vi "Blink_SDK_example_ODP.vi"() -> ()   [LabVIEW 2010]
uses:
  Blink_C_wrapper.dll
  ImageGen.dll
panel:
  in  "True frames":i64=5
  in  "SLM bit depth":u64=8
  out "Boards found":u64
  out "Constructed OK":i64
  in  "Use GPU if available":i64=1
  in  "Maximum Transient Frames":i64=10
  out "Regional LUT File":path
  # "SLM Settings"
  # "These settings should be changed to match your SLM\nbefore running the program."
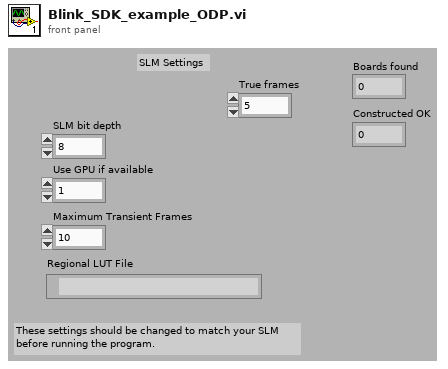
[diagram p1: front panel]
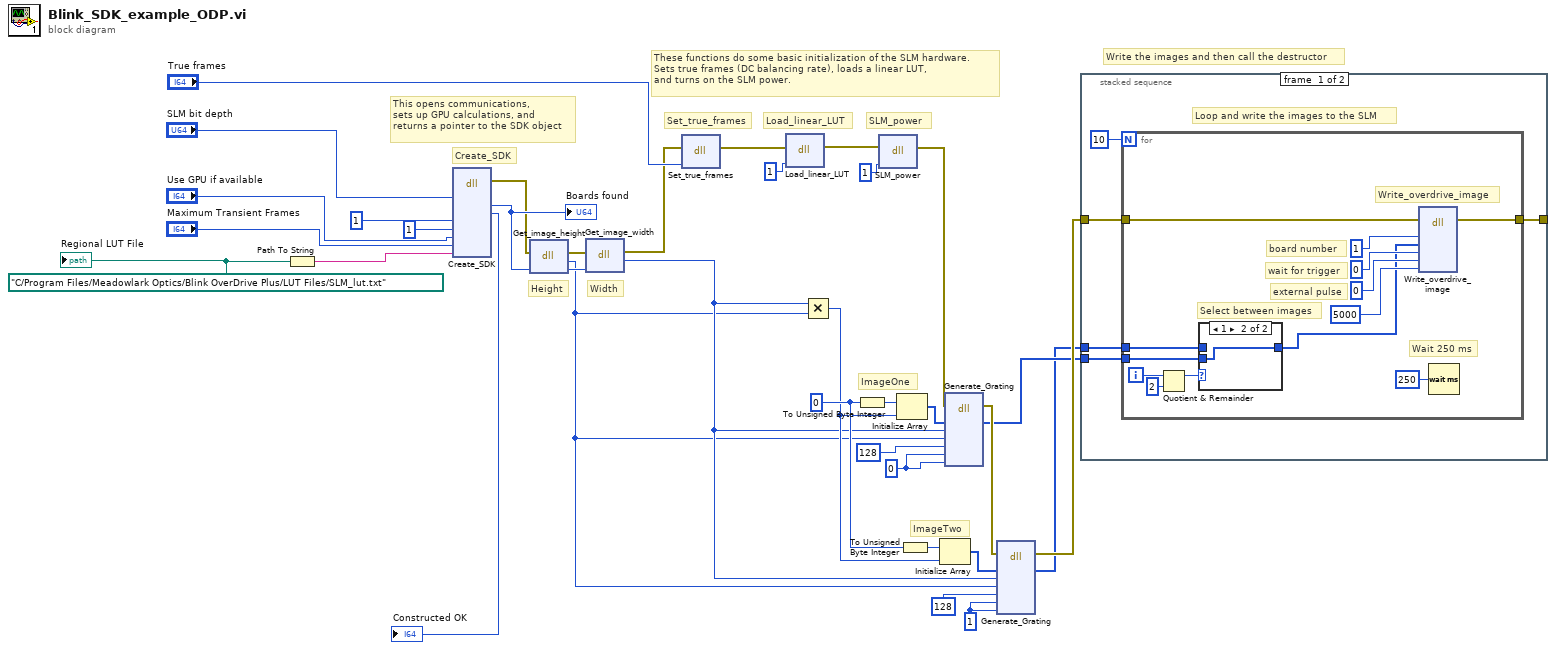
[diagram p0: block diagram]
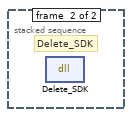
[diagram p3: hidden frame]
diagram:
  w8 = 0
  w11 = 1
  w13 = 0
  w23 = path "C:/Program Files/Meadowlark Optics/Blink OverDrive Plus/LUT Files/SLM_lut.txt" ("path to BMP file")
  # "ImageTwo"
  # "ImageOne"
  # "Width"
  # "Height"
  # "These functions do some basic initialization of the SLM hardware.\nSets true frames (DC balancing rate), loads a linear LUT, \nand turns on the SLM power."
  # "SLM_power"
  # "Load_linear_LUT"
  # "Set_true_frames"
  # "Write the images and then call the destructor"
  # "This opens communications,\nsets up GPU calculations, and\nreturns a pointer to the SDK object"
  # "Create_SDK"
  n1 = Path To String(path=w23) -> (string=w35:string)
  n2 = dll-call lib="C:/Program Files/Meadowlark Optics/Blink OverDrive Plus/SDK/Blink_C_wrapper.dll" fn="Create_SDK"("SLM_bit_depth"="SLM bit depth", "is_nematic_type"=i64 1, "RAM_write_enable"=i64 1, "use_GPU_if_available"="Use GPU if available", "max_transient_frames"="Maximum Transient Frames", "static_regional_lut_file"=w35) -> (error out=w19:errorcluster, "n_boards_found"=w20:u64, "constructed_ok"=→"Constructed OK":i64)  [unwired: 12 in, 1 out]
  "Boards found" <- w20
  n3 = dll-call lib="C:/Program Files/Meadowlark Optics/Blink OverDrive Plus/SDK/Blink_C_wrapper.dll" fn="Get_image_height"(error in=w19, "Board"=w20) -> (error out=w21:errorcluster, "return type"=w5:i32, "Board"=w22:u32)  [unwired: 2 in, 1 out]
  n4 = dll-call lib="C:/Program Files/Meadowlark Optics/Blink OverDrive Plus/SDK/Blink_C_wrapper.dll" fn="Get_image_width"(error in=w21, "Board"=w22) -> (error out=w18:errorcluster, "return type"=w6:i32)  [unwired: 3 in, 1 out]
  n5 = dll-call lib="C:/Program Files/Meadowlark Optics/Blink OverDrive Plus/SDK/Blink_C_wrapper.dll" fn="Set_true_frames"(error in=w18, "true_frames"="True frames") -> (error out=w24:errorcluster)  [unwired: 4 in, 1 out]
  n6 = dll-call lib="C:/Program Files/Meadowlark Optics/Blink OverDrive Plus/SDK/Blink_C_wrapper.dll" fn="Load_linear_LUT"(error in=w24, "board"=i64 1) -> (error out=w25:errorcluster)  [unwired: 4 in, 1 out]
  n7 = Multiply(x=w6, y=w5) -> (x*y=w7:i32)
  n8 = To Unsigned Byte Integer(number=w8) -> (unsigned 8bit integer=w17:u8)
  n9 = dll-call lib="C:/Program Files/Meadowlark Optics/Blink OverDrive Plus/SDK/Blink_C_wrapper.dll" fn="SLM_power"(error in=w25, "power_state"=i64 1) -> (error out=w9:errorcluster)  [unwired: 4 in, 1 out]
  n10 = Initialize Array(w17, w7) -> (w15:u8[])
  n11 = To Unsigned Byte Integer(number=w8) -> (unsigned 8bit integer=w16:u8)
  n12 = Initialize Array(w16, w7) -> (w12:u8[])
  n13 = dll-call lib="C:/Program Files/Meadowlark Optics/Blink OverDrive Plus/SDK/ImageGen.dll" fn="Generate_Grating"(error in=w9, "Array"=w15, "Width"=w6, "Height"=w5, "Period"=128, "Increasing"=w13, "Horizontal"=w13) -> (error out=w4:errorcluster, "Array"=w2:u8[])  [unwired: 8 in, 1 out]
  n14 = dll-call lib="C:/Program Files/Meadowlark Optics/Blink OverDrive Plus/SDK/ImageGen.dll" fn="Generate_Grating"(error in=w4, "Array"=w12, "Width"=w6, "Height"=w5, "Period"=128, "Increasing"=w11, "Horizontal"=w11) -> (error out=w3:errorcluster, "Array"=w1:u8[])  [unwired: 8 in, 1 out]
  n15 = stacked-sequence {
    tunnel: w1 -> [w39 _]
    tunnel: w2 -> [w38 _]
    tunnel: w3 -> [w37 _]
    tunnel: [w36 _] -> _
    frame #0 {
      # "Loop and write the images to the SLM"
      n16 = for {
        N: 10 -> [_]
        tunnel: w39 -> [w47]
        tunnel: w38 -> [w46]
        tunnel: w37 -> [w43]
        tunnel: [w42] -> w36
        i -> [w50]
        # "Wait 250 ms"
        # "Select between images"
        # "external pulse"
        # "wait for trigger"
        # "board number"
        # "Write_overdrive_image"
        n17 = Quotient & Remainder(x=w50, y=2) -> (x-y*floor(x/y)=w48:i32)  [unwired: 1 out]
        n18 = case shown="1" w48 {
          tunnel: w47 -> [w54 _]
          tunnel: w46 -> [_ w55]
          tunnel: [w54 w55] -> w41
          frame 0, Default {
          }
          frame 1 {
          }
        }
        n19 = dll-call lib="C:/Program Files/Meadowlark Optics/Blink OverDrive Plus/SDK/Blink_C_wrapper.dll" fn="Write_overdrive_image"(error in=w43, "board"=i64 1, "target_phase"=w41, "wait_for_trigger"=i64 0, "external_pulse"=i64 0, "Timeout (ms)"=5000) -> (error out=w42:errorcluster)  [unwired: 8 in, 1 out]
        n20 = Wait (ms)(milliseconds to wait=u32 250) -> ()  [unwired: 1 out]
      }
    }
    frame #1 {
      # "Delete_SDK"
      n21 = dll-call lib="C:/Program Files/Meadowlark Optics/Blink OverDrive Plus/SDK/Blink_C_wrapper.dll" fn="Delete_SDK"() -> ()  [unwired: 4 in, 2 out]
    }
  }
  "Regional LUT File" <- w23
